vi "Turret_Aim.vi"(6 "View Button":bool, 7 "Left Trigger":dbl, 8 "Orange Limit Pressed":bool, 9 "Blue Limit Pressed":bool, 10 "Right Bumper":bool, 11 "Left Bumper":bool) -> ()   [LabVIEW 2020]
uses:
  <vilib>/Rock Robotics/WPI/ThirdParty/Phoenix-LabVIEW/Motor Controller/Controls/CTRE_Phoenix_MotorControl_ControlMode.ctl
  <vilib>/Rock Robotics/WPI/ThirdParty/Phoenix-LabVIEW/Motor Controller/Get/CTRE_Phoenix_MotorController_IntegratedSensorData_TalonFX.vi
  <vilib>/Rock Robotics/Network Tables/NT Read Number.vi
  <vilib>/addons/control/pid/pid.llb/PID (DBL).vi
  <vilib>/Rock Robotics/Network Tables/NT Write Number.vi
  <vilib>/addons/control/pid/NI_PID_pid.lvlib
panel:
  in  "setpoint":dbl=-2.0 format="%#_13g"
  out "Ty":dbl
  out "Tx":dbl
  in  "Turret Auto Aim PID":T1={"proportional gain (Kc)"=-0.015, "integral time (Ti, min)"=0.0, "derivative time (Td, min)"=5e-05} {"derivative time (Td, min)" format="%.6f"; "integral time (Ti, min)" format="%.3f"; "proportional gain (Kc)" format="%.3f"}
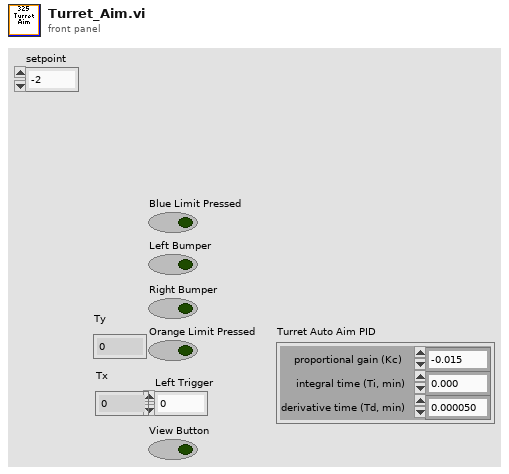
[diagram p1: front panel]
types:
  T1 = cluster{"proportional gain (Kc)":dbl, "integral time (Ti, min)":dbl, "derivative time (Td, min)":dbl}
  T2 = typedef "WPI_MotorControlDeviceRef.ctl" = cluster{"DeviceStatus":errorcluster, "Type":T3, "PWM":cluster{"PWM Channel":T4, "DeadBand":T5}, "CAN":cluster{"Device Number":u8, "SetOutput VI Ref":variant, "GetOutput VI Ref":variant, "Enable VI Ref":variant, "Disable VI Ref":variant, "Data":variant}, "Invert":bool, "DIO PWM":cluster{"PWM \"Enable\" Channel":T4, "DIOChannel":T6, "PWM Rate":dbl}}
  T3 = typedef "WPI_MotorControlType.ctl" = enum16{"PWM", "CAN", "DIO PWM"}
  T4 = typedef "FPGA_DIOPWMChannel.ctl" = enum8{"PWM 0", "PWM 1", "PWM 2", "PWM 3", "PWM 4", "PWM 5", "PWM 6", "PWM 7", "PWM 8", "PWM 9", "PWM MXP 0", "PWM MXP 1", "PWM MXP 2", "PWM MXP 3", "PWM MXP 4", "PWM MXP 5", "PWM MXP 6", "PWM MXP 7", "PWM MXP 8", "PWM MXP 9", "Invalid"}
  T5 = typedef "WPI_PWMDeadband.ctl" = cluster{"Name":string, "maxPositivePwm":i32, "minPositivePwm":i32, "centerPwm":i32, "maxNegativePwm":i32, "minNegativePwm":i32, "angularRange":u16}
  T6 = typedef "FPGA_DIOChannel.ctl" = enum8{"DIO 0", "DIO 1", "DIO 2", "DIO 3", "DIO 4", "DIO 5", "DIO 6", "DIO 7", "DIO 8", "DIO 9", "DIO MXP 0", "DIO MXP 1", "DIO MXP 2", "DIO MXP 3", "DIO MXP 4", "DIO MXP 5", "DIO MXP 6", "DIO MXP 7", "DIO MXP 8", "DIO MXP 9", "DIO MXP 10", "DIO MXP 11", "DIO MXP 12", "DIO MXP 13", "DIO MXP 14", "DIO MXP 15", "SPI Port CS1", "SPI Port CS2", "SPI Port CS3", "SPI Port MISO", "SPI Port MOSI", "Invalid"}
  T7 = typedef "CTRE_Phoenix_MotorControl_ControlMode.ctl" = u16
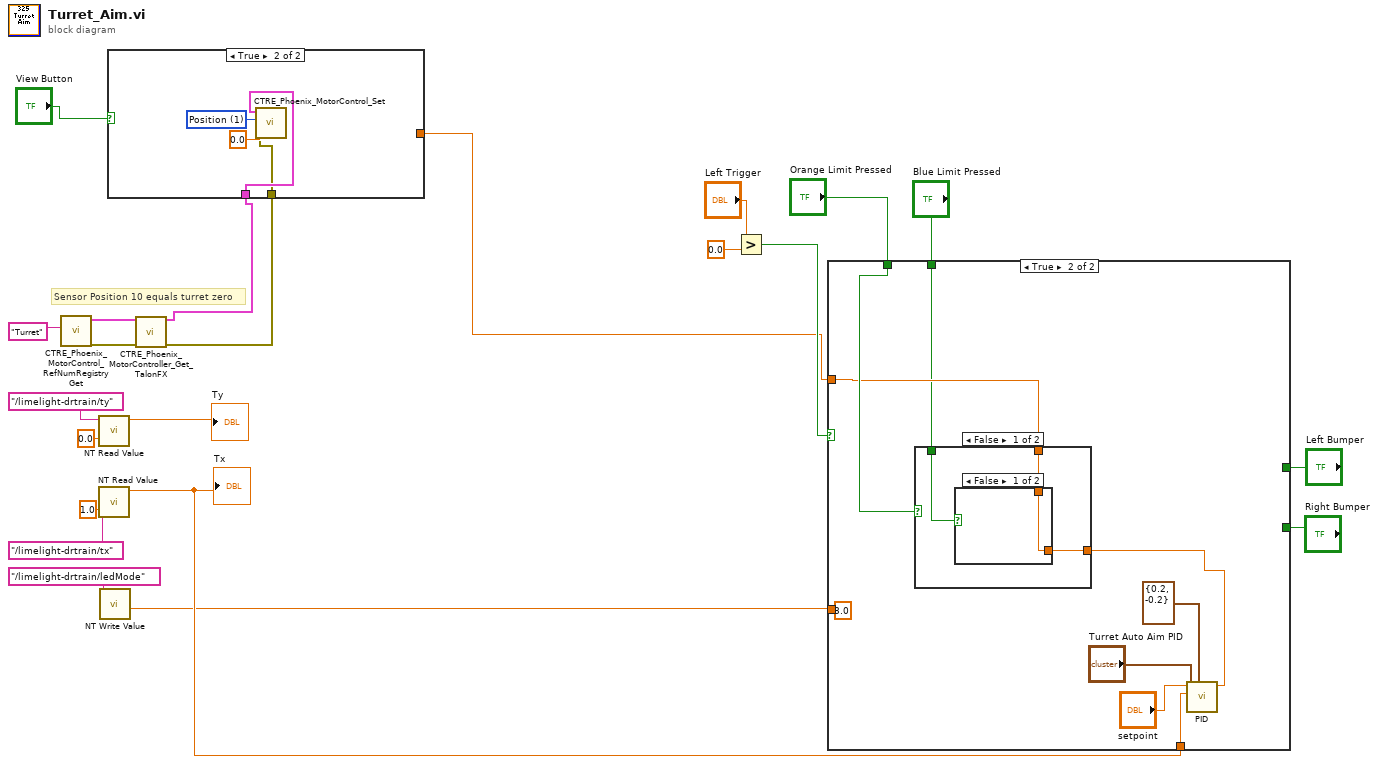
[diagram p0: block diagram]
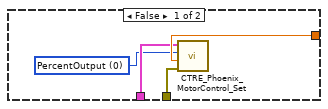
[diagram p2: hidden frame]
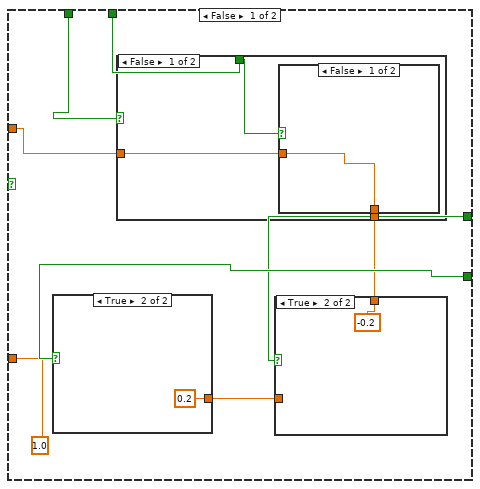
[diagram p3: hidden frame]
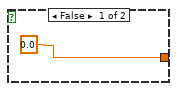
[diagram p5: hidden frame]
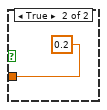
[diagram p6: hidden frame]
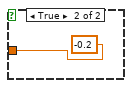
[diagram p7: hidden frame]
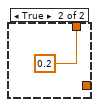
[diagram p8: hidden frame]
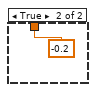
[diagram p9: hidden frame]
diagram:
  # "Sensor Position 10 equals turret zero"
  n1 = call <vilib>:"CTRE_Phoenix_MotorControl_RefNumRegistryGet.vi"("refnum name"="Turret") -> ("error out"=w6:errorcluster, "PhoenixMotorControlDevRef"=w14:T2)  [unwired: 9 in]
  n2 = call-poly <vilib>:"NT Read Value.vi"("Default Value"=0.0, "Name"="/limelight-drtrain/ty") -> ("Numeric"=→"Ty":dbl)  [unwired: 8 in, 1 out]
  n3 = call-poly <vilib>:"NT Read Value.vi"("Default Value"=1.0, "Name"="/limelight-drtrain/tx") -> ("Numeric"=w8:dbl)  [unwired: 8 in, 1 out]
  "Tx" <- w8
  n4 = call-poly <vilib>:"CTRE_Phoenix_MotorController_Get_TalonFX.vi"("PhoenixMotorControlDevRef"=w14, "error in"=w6) -> ("PhoenixMotorControlDevRef"=w4:T2, "error out"=w5:errorcluster)  [unwired: 9 in, 3 out]
  n5 = Greater?(x="Left Trigger", y=0.0) -> (0:w7:bool)
  n6 = case shown="True" w7 {
    tunnel: [w24 w45] -> w2
    tunnel: "Orange Limit Pressed" -> [w30 w46]
    tunnel: "Blue Limit Pressed" -> [w29 w43]
    tunnel: "Right Bumper" -> [w28 _]
    tunnel: "Left Bumper" -> [w27 _]
    tunnel: [1.0 ("Numeric") 3.0 ("ledMode")] -> w3
    tunnel: w8 -> [_ w41]
    frame False {
      n7 = case shown="True" w28 {
        tunnel: [0.0 ("output") 0.2 ("output")] -> w26
        frame False {
        }
        frame True {
        }
      }
      n8 = case shown="True" w27 {
        tunnel: w26 -> [w31 _]
        tunnel: [w31 -0.2 ("output")] -> w25
        frame False {
        }
        frame True {
        }
      }
      n9 = case shown="False" w30 {
        tunnel: w29 -> [w37 _]
        tunnel: w25 -> [w36 _]
        tunnel: [w35 -0.2 ("output")] -> w24
        frame False {
          n10 = case shown="False" w37 {
            tunnel: w36 -> [w38 _]
            tunnel: [w38 0.2 ("output")] -> w35
            frame False {
            }
            frame True {
            }
          }
        }
        frame True {
        }
      }
    }
    frame True {
      n11 = call-poly <vilib>:"PID.vi"("output range"=cluster{"output high":dbl, "output low":dbl} {"output high"=0.2, "output low"=-0.2}, "PID gains"="Turret Auto Aim PID", "process variable"=w41, "setpoint"="setpoint") -> ("output"=w44:dbl)  [unwired: 6 in, 1 out]
      n12 = case shown="False" w46 {
        tunnel: [w51 -0.2 ("output")] -> w45
        tunnel: w44 -> [w50 _]
        tunnel: w43 -> [w52 _]
        frame False {
          n13 = case shown="False" w52 {
            tunnel: [w53 0.2 ("output")] -> w51
            tunnel: w50 -> [w53 _]
            frame False {
            }
            frame True {
            }
          }
        }
        frame True {
        }
      }
    }
  }
  n14 = call-poly <vilib>:"NT Write Value.vi"("Numeric"=w3, "Name"="/limelight-drtrain/ledMode") -> ()  [unwired: 9 in, 1 out]
  n15 = case shown="True" "View Button" {
    tunnel: w5 -> [w59 w60]
    tunnel: w2 -> [w58 _]
    tunnel: w4 -> [w57 w61]
    frame False {
      w56 = T7 0 items=["PercentOutput"=0, "Position"=1, "Velocity"=2, "Current"=3, "Follower"=5, "MotionProfile"=6, "MotionMagic"=7, "MotionProfileArc"=10, "Disabled"=15] ("Control Mode")
      n16 = call <vilib>:"CTRE_Phoenix_MotorControl_Set.vi"("error in (no error)"=w59, "Output"=w58, "Control Mode"=w56, "PhoenixMotorControlDevRef"=w57) -> ()  [unwired: 6 in, 2 out]
    }
    frame True {
      w63 = T7 1 items=["PercentOutput"=0, "Position"=1, "Velocity"=2, "Current"=3, "Follower"=5, "MotionProfile"=6, "MotionMagic"=7, "MotionProfileArc"=10, "Disabled"=15] ("Control Mode")
      n17 = call <vilib>:"CTRE_Phoenix_MotorControl_Set.vi"("error in (no error)"=w60, "Output"=0.0, "Control Mode"=w63, "PhoenixMotorControlDevRef"=w61) -> ()  [unwired: 6 in, 2 out]
    }
  }
